vi "setStyle.vi"(8 "error in (no error)":errorcluster, 10 "Style":refnum<class "Style.lvclass">, 11 "MS-Excel in":refnum<class "MS-Excel.lvclass">) -> (0 "error out":errorcluster, 3 "MS-Excel out":refnum<class "MS-Excel.lvclass">)   [LabVIEW 2020, in "LabVIEW NPOI.lvlib" / "MS-Excel.lvclass"]
uses:
  MS-Excel.lvclass
  Styles/Style/Style.lvclass
  MS-Excel.lvclass/MS-Excel.ctl
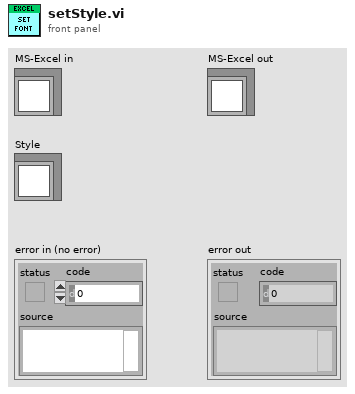
[diagram p1: front panel]
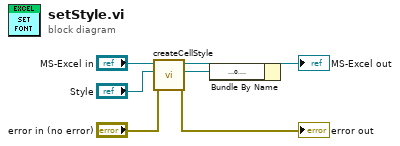
[diagram p0: block diagram]
diagram:
  n1 = call-dynamic "createCellStyle.vi"("error in (no error)"="error in (no error)", "Style"="Style", "MS-Excel in"="MS-Excel in") -> ("error out"=→"error out":errorcluster, "Cell Style"=w1:refnum<k24>, "MS-Excel out"=w4:refnum<class "MS-Excel.lvclass">)  [unwired: 6 in]
  n2 = Bundle By Name(cluster=w4, "Cell Style"=w1) -> (→"MS-Excel out":refnum<class "MS-Excel.lvclass">)
